vi "Excel_DA_ Remainder.vi"(3 "DA":dbl=1.125, 5 "Value":dbl) -> (0 "Column":i32, 1 "remainder":dbl format="%#.6g", 2 "x > 0?":bool)   [LabVIEW 2015]
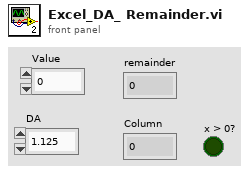
[diagram p1: front panel]
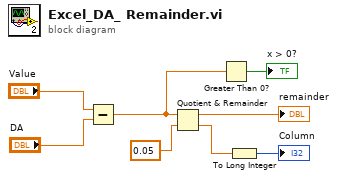
[diagram p0: block diagram]
diagram:
  n1 = Subtract(x="Value", y="DA") -> (x-y=w2:dbl)
  n2 = Quotient & Remainder(x=w2, y=0.05) -> (x-y*floor(x/y)=→"remainder":dbl, floor(x/y)=w6:dbl)
  n3 = Greater Than 0?(x=w2) -> (x > 0?=→"x > 0?":bool)
  n4 = To Long Integer(number=w6) -> (32bit integer=→"Column":i32)
